vi "SVT UFF58 Write Record 10.vi"(0 "function refnum":refnum<k20>, 5 "ordinate denominator data characteristics":T1 {"specific data type" items=["unknown"=0, "general"=1, "stress"=2, "strain"=3, "temperature"=5, "heat flux"=6, "displacement"=8, "reaction force"=9, "velocity"=11, "acceleration"=12, "excitation force"=13, "pressure"=15, "mass"=16, "time"=17, "frequency"=18, "rpm"=19, "order"=20, "sound pressure"=21, "sound intensity"=22, "sound power"=23]}, 11 "error in (no error)":errorcluster) -> (4 "dup function refnum":refnum<k20>, 15 "error out":errorcluster)   [LabVIEW 2017, in "SoundVib_UFF58.lvlib"]
doc: "Writes the values of the fields in record 10 of the UFF58 (universal file format) file. Record 10 contains the ordinate denominator data characteristics. Record 9 contains the ordinate or ordinate numerator data characteristics. Use this VI with the SVT UFF58 Write Record 9 VI if you need to write ordinate denominator and ordinate numerator characteristics."
uses:
  <vilib>/addons/Sound and Vibration/svt_UFF58/SoundVib_UFF58.lvlib
  <vilib>/addons/Sound and Vibration/svt_UFF58/subVIs/sv_UFF58 Axis Characteristics.ctl
  <vilib>/addons/Sound and Vibration/svt_UFF58/subVIs/sv_UFF58 Specific Datatype.ctl
  <vilib>/Platform/storage/Storage.llb/Set Property (String).vi
  <vilib>/Platform/storage/Storage.llb/Set Property (I32).vi
  <vilib>/Platform/storage/Storage.llb/Get Property (Storage Refnums).vi
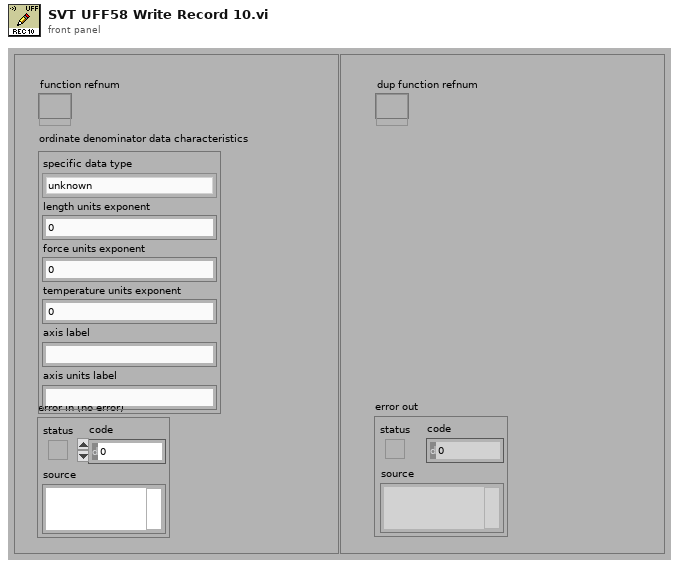
[diagram p1: front panel]
types:
  T1 = typedef "SoundVib_UFF58.lvlib/sv_UFF58 Axis Characteristics.ctl" = cluster{"specific data type":T2, "length units exponent":i32, "force units exponent":i32, "temperature units exponent":i32, "axis label":string, "axis units label":string}
  T2 = typedef "SoundVib_UFF58.lvlib/sv_UFF58 Specific Datatype.ctl" = u16
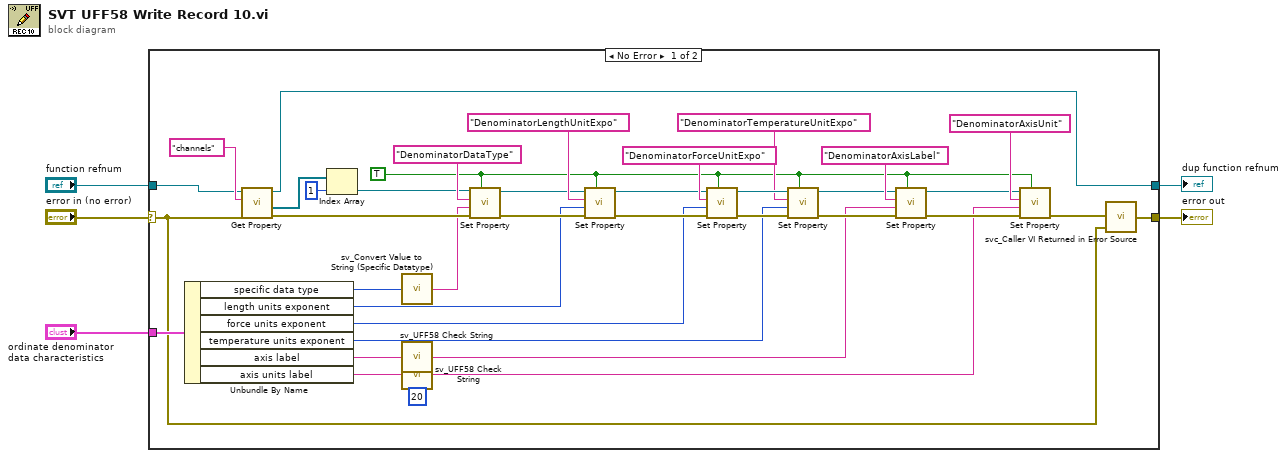
[diagram p0: block diagram]
diagram:
  n1 = case shown="No Error" "error in (no error)" {
    selector: "error in (no error)" -> [w9 w44]
    tunnel: [w11 w44] -> w5
    tunnel: "ordinate denominator data characteristics" -> [w25 _]
    tunnel: "function refnum" -> [w14 w45]
    tunnel: [w13 w45] -> w1
    frame No Error {
      w8 = TRUE ("User-defined property")
      w12 = 20 ("length (rest)")
      n2 = Unbundle By Name(w25) -> ("specific data type"=w7:T2, "length units exponent"=w24:i32, "force units exponent"=w23:i32, "temperature units exponent"=w22:i32, "axis label"=w26:string, "axis units label"=w27:string)
      n3 = call-poly <vilib>:"Get Property.vi"("error in (no error)"=w9, "Property name"="channels", "storage refnum"=w14) -> ("error out"=w16:errorcluster, "Value"=w18:refnum<k20>[], "storage refnum out"=w13:refnum<k20>)  [unwired: 6 in]
      n4 = Index Array(array=w18, index=1) -> (element=w15:refnum<k20>)
      n5 = call <vilib>:"sv_Convert Value to String (Specific Datatype).vi"("specific data type value"=w7) -> ("specific data type string"=w6:string)  [unwired: 14 in]
      n6 = call <vilib>:"sv_UFF58 Check String.vi"("field value"=w26, "field length"=w12) -> ("output string"=w21:string)  [unwired: 12 in, 1 out]
      n7 = call <vilib>:"sv_UFF58 Check String.vi"("field value"=w27, "field length"=w12) -> ("output string"=w20:string)  [unwired: 12 in, 1 out]
      n8 = call-poly <vilib>:"Set Property.vi"("Create if not found (no:F)"=w8, "error in (no error)"=w16, "Value"=w6, "Property name"="DenominatorDataType", "storage refnum"=w15) -> ("error out"=w40:errorcluster, "storage refnum out"=w39:refnum<k20>)  [unwired: 5 in]
      n9 = call-poly <vilib>:"Set Property.vi"("Create if not found (no:F)"=w8, "error in (no error)"=w40, "Value"=w24, "Property name"="DenominatorLengthUnitExpo", "storage refnum"=w39) -> ("error out"=w36:errorcluster, "storage refnum out"=w37:refnum<k20>)  [unwired: 5 in]
      n10 = call-poly <vilib>:"Set Property.vi"("Create if not found (no:F)"=w8, "error in (no error)"=w36, "Value"=w23, "Property name"="DenominatorForceUnitExpo", "storage refnum"=w37) -> ("error out"=w34:errorcluster, "storage refnum out"=w35:refnum<k20>)  [unwired: 5 in]
      n11 = call-poly <vilib>:"Set Property.vi"("Create if not found (no:F)"=w8, "error in (no error)"=w34, "Value"=w22, "Property name"="DenominatorTemperatureUnitExpo", "storage refnum"=w35) -> ("error out"=w30:errorcluster, "storage refnum out"=w31:refnum<k20>)  [unwired: 5 in]
      n12 = call-poly <vilib>:"Set Property.vi"("Create if not found (no:F)"=w8, "error in (no error)"=w30, "Value"=w21, "Property name"="DenominatorAxisLabel", "storage refnum"=w31) -> ("error out"=w28:errorcluster, "storage refnum out"=w29:refnum<k20>)  [unwired: 5 in]
      n13 = call-poly <vilib>:"Set Property.vi"("Create if not found (no:F)"=w8, "error in (no error)"=w28, "Value"=w20, "Property name"="DenominatorAxisUnit", "storage refnum"=w29) -> ("error out"=w10:errorcluster)  [unwired: 5 in, 1 out]
      n14 = call <vilib>:"svc_Caller VI Returned in Error Source.vi"("warning input to caller"=w9, "error in (no error)"=w10) -> ("error out"=w11:errorcluster)  [unwired: 3 in]
    }
    frame Error {
    }
  }
  "error out" <- w5
  "dup function refnum" <- w1
